vi "Collection.vi"(8 "error in (no error)":errorcluster, 11 "Node Ptr":T1 format="%.0x") -> (0 "error out":errorcluster)   [LabVIEW 2015, in "Diagnostics Addon System Explorer.lvlib"]
uses:
  Diagnostics Addon System Explorer.lvlib
  <vilib>/NI Veristand/Custom Device API/Custom Device Item Ref.ctl
  Types/FG.Action.ctl
  Shared/SubVIs/Constants.vi
  <vilib>/NI/NIVS System Definition Utilities/SysDef API/SysDef.Property.Set.vi
  <vilib>/NI/NIVS System Definition Utilities/_SubVIs/SysDef.Property.Set.U32.vi
  <vilib>/NI Veristand/Custom Device API/NI VeriStand - Get Item Property.vi
  <vilib>/NI Veristand/Custom Device API/Get Item Property (U32).vi
  <vilib>/NI Veristand/Custom Device API/Custom Device API.lvlib
panel:
  in  "ID":u16 format="%.0x"
  in  "Description":string
  in  "Name":string
  in  "SHDocVw.IWebBrowser":refnum<k7>(container)
  in  "Header":cluster{"Section Name":string}={"Section Name"="Custom Device Item Settings"}
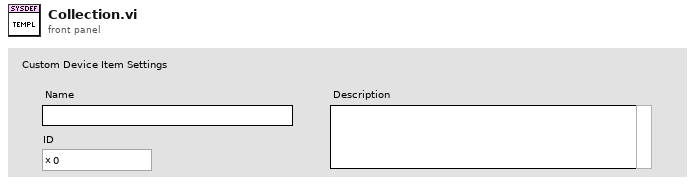
[diagram p1: front panel]
types:
  T1 = typedef "Custom Device API.lvlib/Custom Device Item Ref.ctl" = u64
  T2 = typedef "Diagnostics Addon System Explorer.lvlib/FG.Action.ctl" = enum16{"Get", "Set"}
  T3 = typedef "Custom Device API.lvlib/Custom Device Item Info.ctl" = cluster{"Name":string, "Is Channel":bool, "GUID":string, "Is Waveform":bool}
  T4 = typedef "Custom Device API.lvlib/Custom Device Commands.ctl" = enum16{"Default", "Item renamed", "Shutdown", "Dynamic button pressed"}
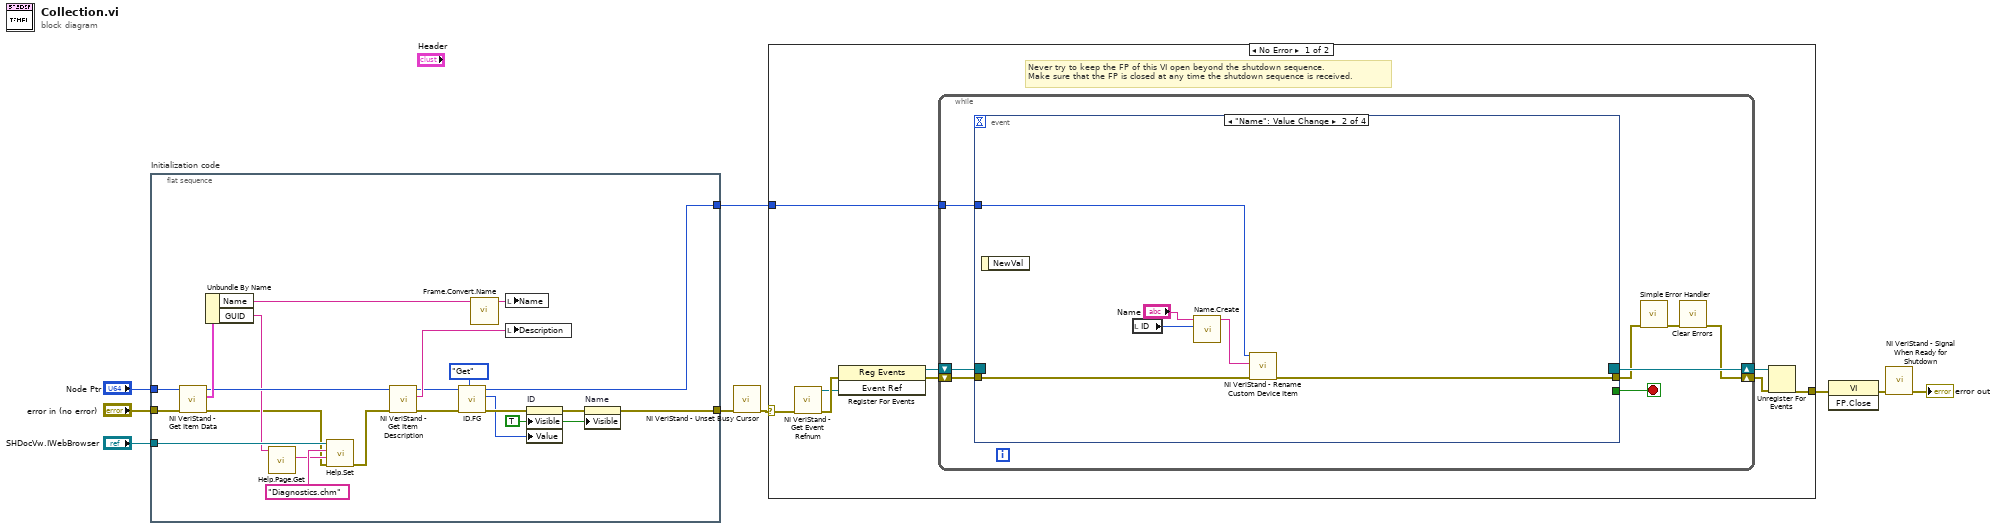
[diagram p0: block diagram]
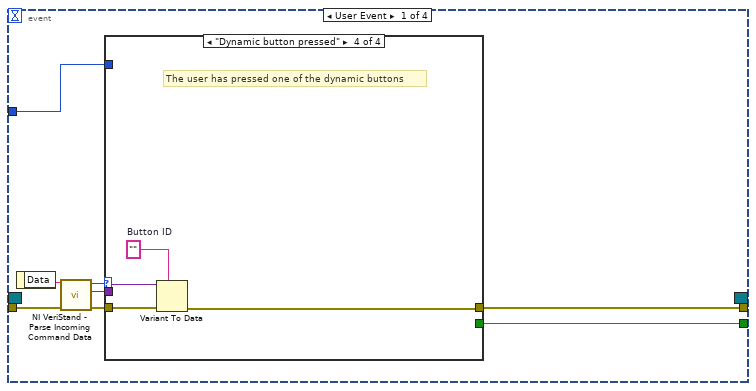
[diagram p2: hidden frame]
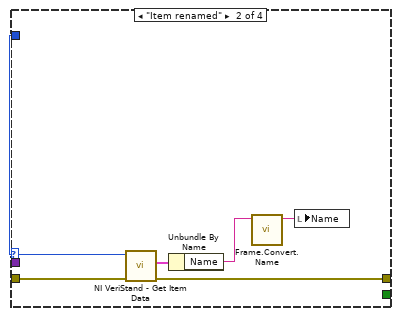
[diagram p4: hidden frame]
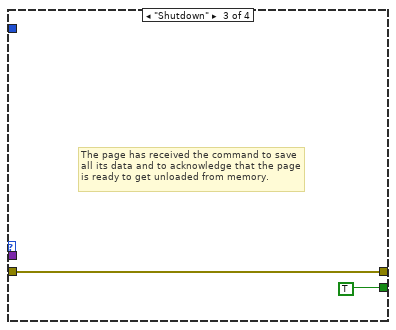
[diagram p5: hidden frame]
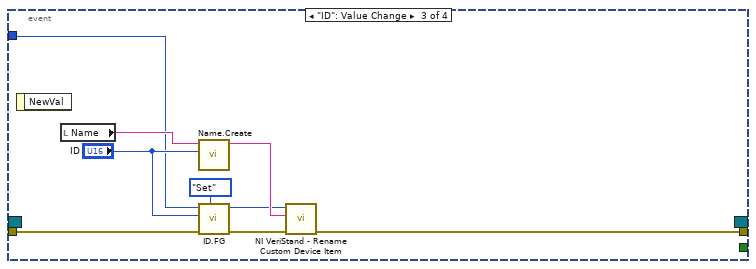
[diagram p6: hidden frame]
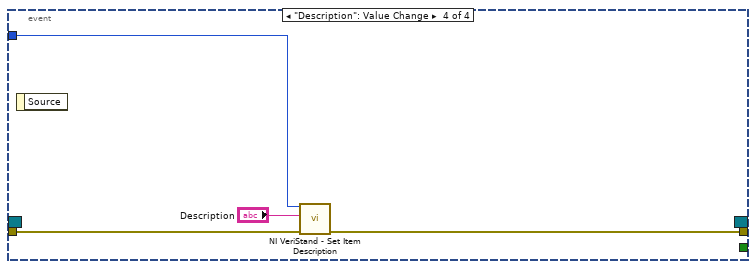
[diagram p7: hidden frame]
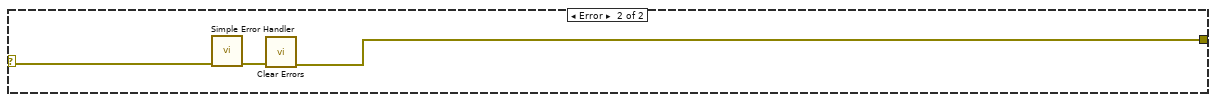
[diagram p8: hidden frame]
diagram:
  n1 = flat-sequence "Initialization code" {
    tunnel: "error in (no error)" -> [w13]
    tunnel: "Node Ptr" -> [w23]
    tunnel: [w15] -> w5
    tunnel: [w21] -> w2
    tunnel: "SHDocVw.IWebBrowser" -> [w22]
    frame #0 {
      w16 = TRUE ("Visible")
      n2 = call <vilib>:"NI VeriStand - Get Item Data.vi"("error in (no error)"=w13, "Item Ref in"=w23) -> ("error out"=w11:errorcluster, "Item Info"=w30:T3, "Item Ref out"=w24:T1)  [unwired: 7 out]
      n3 = Unbundle By Name(w30) -> ("Name"=w28:string, "GUID"=w12:string)
      n4 = call "Help.Page.Get.vi"("GUID"=w12) -> ("HTML File"=w14:string)  [unwired: 10 in]
      n5 = call "Help.Set.vi"("error in (no error)"=w11, "HTML File"=w14, "Main CHM File"="Diagnostics.chm", "SHDocVw.IWebBrowser2"=w22) -> ("error out"=w10:errorcluster)  [unwired: 7 in]
      n6 = call <vilib>:"NI VeriStand - Get Item Description.vi"("error in (no error)"=w10, "Item Ref in"=w24) -> ("error out"=w26:errorcluster, "Description"=w31:string, "Item Ref out"=w25:T1)  [unwired: 7 out]
      n7 = call "ID.FG.vi"("Action"=FG.Action."Get", "error in (no error)"=w26, "Device Item Ref in"=w25) -> ("error out"=w19:errorcluster, "ID"=w18:u32, "Device Item Ref out"=w21:T1)  [unwired: 6 in]
      n8 = call "Frame.Convert.Name.vi"("VS Frame Name"=w28) -> ("Frame Name"=w27:string)  [unwired: 9 in, 1 out]
      n9 = local write "Name"(w27) -> ()
      n10 = local write "Description"(w31) -> ()
      n11 = property on="ID" class="DigNum (strict)"(error in=w19, "Visible"=w16, "Value"=w18) -> (error out=w17:errorcluster)  [unwired: 1 in, 1 out]
      n12 = property on="Name" class="Str"(error in=w17, "Visible"=w16) -> (error out=w15:errorcluster)  [unwired: 1 in, 1 out]
    }
  }
  n13 = call <vilib>:"NI VeriStand - Unset Busy Cursor.vi"("error in (no error)"=w5) -> ("error out"=w4:errorcluster)  [unwired: 10 out]
  n14 = case shown="No Error" w4 {
    selector: w4 -> [w32 w91]
    tunnel: [w37 w89] -> w9
    tunnel: w2 -> [w33 _]
    frame No Error {
      # "Never try to keep the FP of this VI open beyond the shutdown sequence.\nMake sure that the FP is closed at any time the shutdown sequence is received."
      n15 = call <vilib>:"NI VeriStand - Get Event Refnum.vi"("error in (no error)"=w32) -> ("error out"=w40:errorcluster, "Event Ref"=w36:refnum<user-event>)  [unwired: 9 out]
      n16 = register-events(error in=w40, w36) -> (reference out=w34:refnum<event-registration>, error out=w35:errorcluster)  [unwired: 1 in]
      n17 = while {
        tunnel: w33 -> [w44]
        shift-right: [w41] -> w38
        shift-left: w35 -> [w47]
        shift-right: [w48] -> w39
        shift-left: w34 -> [w46]
        stop <- w45 stop-if-true
        n18 = event shown="[1] \"Name\": Value Change" {
          selector: w46 -> [_ _ _ _]
          dyn-events: [_ _ _ _] -> w48
          timeout: _ -> [_ _ _ _]
          tunnel: w47 -> [w56 w75 w81 w87]
          tunnel: [w52 _ _ _] -> w45
          tunnel: [w51 w74 w83 w86] -> w43
          tunnel: w44 -> [w50 w73 w78 w88]
          event User Event {
            n19 = event-data() -> ("Data"=w55:string)  [unwired: 1 out]
            n20 = call <vilib>:"NI VeriStand - Parse Incoming Command Data.vi"("error in (no error)"=w56, "Incoming data"=w55) -> ("error out"=w54:errorcluster, "Outgoing data"=w49:variant, "Action"=w53:T4)  [unwired: 7 out]
            n21 = case shown="\"Dynamic button pressed\"" w53 {
              tunnel: w54 -> [w57 w63 w64 w69]
              tunnel: [_ _ TRUE _] -> w52
              tunnel: [w57 w60 w64 w66] -> w51
              tunnel: w50 -> [_ w62 _ _]
              tunnel: w49 -> [_ _ _ w68]
              frame "Default", Default {
              }
              frame "Item renamed" {
                n22 = call <vilib>:"NI VeriStand - Get Item Data.vi"("error in (no error)"=w63, "Item Ref in"=w62) -> ("error out"=w60:errorcluster, "Item Info"=w61:T3)  [unwired: 8 out]
                n23 = Unbundle By Name(w61) -> ("Name"=w59:string)
                n24 = call "Frame.Convert.Name.vi"("VS Frame Name"=w59) -> ("Frame Name"=w58:string)  [unwired: 9 in, 1 out]
                n25 = local write "Name"(w58) -> ()
              }
              frame "Shutdown" {
                # "The page has received the command to save all its data and to acknowledge that the page is ready to get unloaded from memory."
              }
              frame "Dynamic button pressed" {
                w67 = ""  # Button ID
                # "The user has pressed one of the dynamic buttons"
                n26 = Variant To Data(error in=w69, type=w67, Variant=w68) -> (error out=w66:errorcluster)  [unwired: 1 out]
              }
            }
          }
          event "Name": Value Change {
            n27 = event-data() -> ()  [unwired: 2 out]
            n28 = local read "ID"() -> (w72:u16)
            n29 = call "Name.Create.vi"("PID Number"=w72, "PID Name"="Name") -> ("VS Name"=w70:string)  [unwired: 9 in]
            n30 = call <vilib>:"NI VeriStand - Rename Custom Device Item.vi"("error in (no error)"=w75, "New Name"=w70, "Item Ref in"=w73) -> ("error out"=w74:errorcluster)  [unwired: 1 in, 7 out]
          }
          event "ID": Value Change {
            n31 = event-data() -> ()  [unwired: 2 out]
            n32 = local read "Name"() -> (w82:string)
            n33 = call "Name.Create.vi"("PID Number"="ID", "PID Name"=w82) -> ("VS Name"=w84:string)  [unwired: 9 in]
            n34 = call "ID.FG.vi"("Action"=FG.Action."Set", "error in (no error)"=w81, "ID"="ID", "Device Item Ref in"=w78) -> ("error out"=w80:errorcluster, "Device Item Ref out"=w77:T1)  [unwired: 5 in, 1 out]
            n35 = call <vilib>:"NI VeriStand - Rename Custom Device Item.vi"("error in (no error)"=w80, "New Name"=w84, "Item Ref in"=w77) -> ("error out"=w83:errorcluster)  [unwired: 1 in, 7 out]
          }
          event "Description": Value Change {
            n36 = event-data() -> ()  [unwired: 2 out]
            n37 = call <vilib>:"NI VeriStand - Set Item Description.vi"("error in (no error)"=w87, "Description"="Description", "Item Ref in"=w88) -> ("error out"=w86:errorcluster)  [unwired: 8 out]
          }
        }
        n38 = call <vilib>:"Simple Error Handler.vi"("error in (no error)"=w43) -> ("error out"=w42:errorcluster)  [unwired: 1 in, 7 out]
        n39 = call <vilib>:"Clear Errors.vi"("error in (no error)"=w42) -> ("error out"=w41:errorcluster)  [unwired: 1 in, 5 out]
      }
      n40 = Unregister For Events(event registration refnum=w39, error in=w38) -> (error out=w37:errorcluster)
    }
    frame Error {
      n41 = call <vilib>:"Simple Error Handler.vi"("error in (no error)"=w91) -> ("error out"=w90:errorcluster)  [unwired: 1 in, 7 out]
      n42 = call <vilib>:"Clear Errors.vi"("error in (no error)"=w90) -> ("error out"=w89:errorcluster)  [unwired: 1 in, 5 out]
    }
  }
  n43 = invoke class="VI" method="FP.Close"(error in=w9) -> (error out=w8:errorcluster)  [unwired: 2 in, 2 out]
  n44 = call <vilib>:"NI VeriStand - Signal When Ready for Shutdown.vi"("error in (no error)"=w8) -> ("error out"=→"error out":errorcluster)  [unwired: 10 out]
